vi "write data.vi"(8 "error in":errorcluster, 9 "timeout":i32=-1, 10 "data":string, 11 "lvlibretls connection in":refnum<class "lvlibretls connection.lvclass">) -> (0 "error out":errorcluster, 3 "lvlibretls connection out":refnum<class "lvlibretls connection.lvclass">)   [LabVIEW 2016, in "lvlibretls connection.lvclass"]
doc: "Writes all data to the network. Internally takes several attempts because libtls accepts only ~16 kB at a time (probably machine dependent). Trying to write a huge file will result in (a) many attempts, which could induce data copies, and (b) multiple \"string subset\" calls. Keeping writes under 10 kB where reasonable is a good idea unless you've really just got one big chunk of data (like an image). If you can process in smaller chunks (like sending a file off disk) you will probably see performance improvements from doing this."
uses:
  lvlibretls connection.lvclass
  lvlibretls connection.lvclass/lvlibretls connection.ctl
  tls library paths.vi
  lv tls dll.lvlib
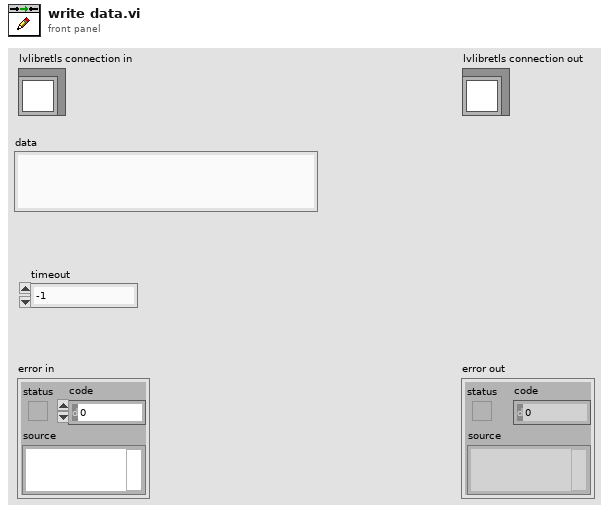
[diagram p1: front panel]
types:
  T1 = enum16{"Standard", "Buffered", "CRLF", "Immediate"}
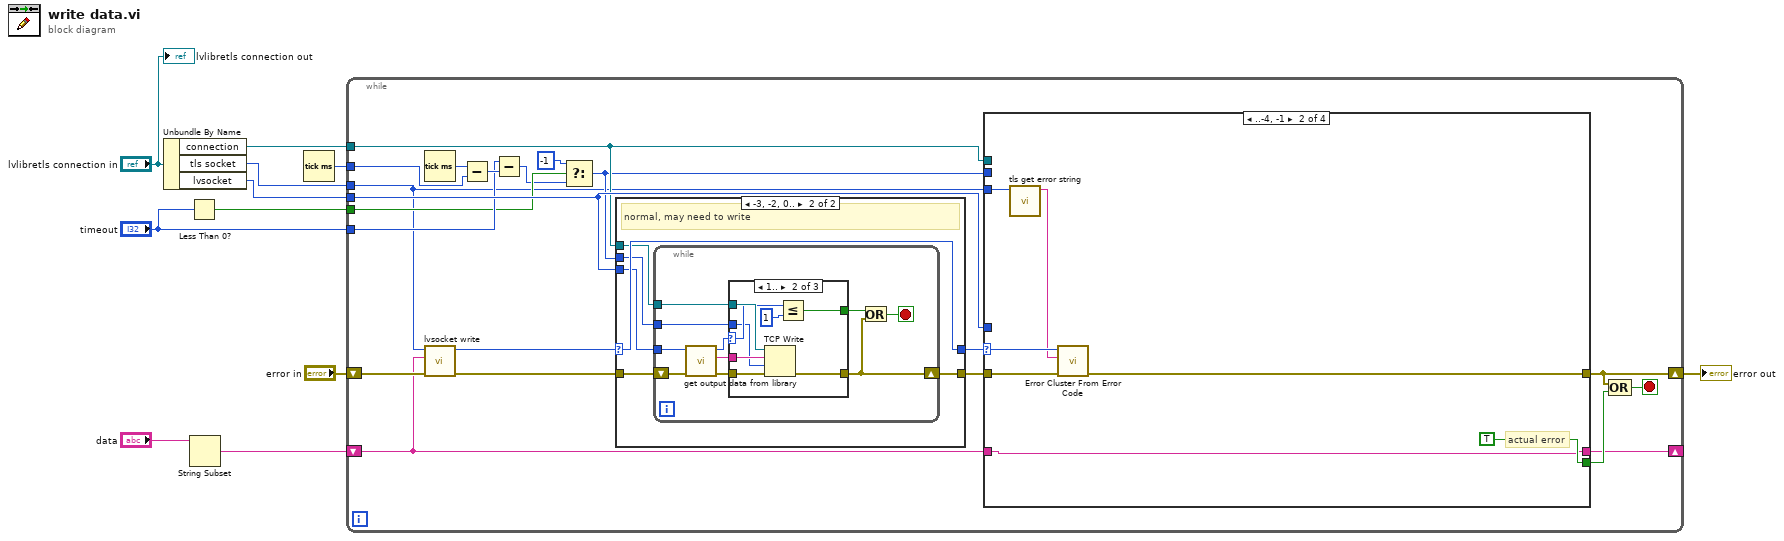
[diagram p0: block diagram]
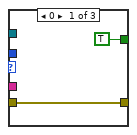
[diagram p3: hidden frame]
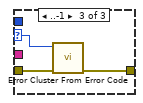
[diagram p4: hidden frame]
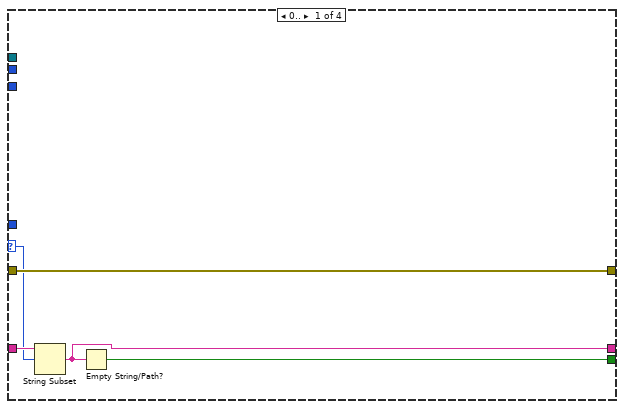
[diagram p5: hidden frame]
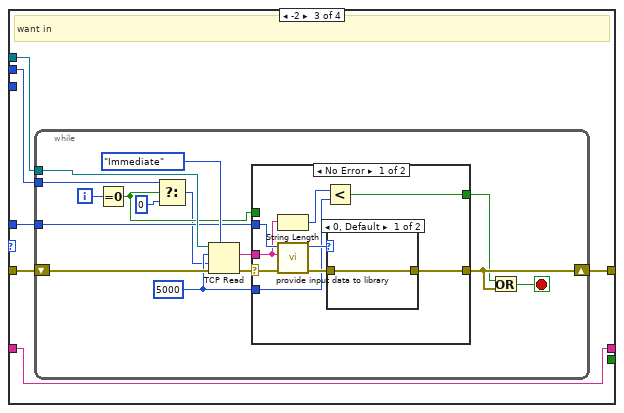
[diagram p6: hidden frame]
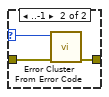
[diagram p7: hidden frame]
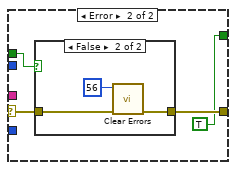
[diagram p8: hidden frame]
diagram:
  n1 = Unbundle By Name("lvlibretls connection in") -> ("connection"=w9:refnum<k5>, "tls socket"=w10:u64, "lvsocket"=w8:u64)
  n2 = Less Than 0?(x="timeout") -> (x < 0?=w4:bool)
  n3 = String Subset(string="data") -> (substring=w1:string)  [unwired: 2 in]
  n4 = Tick Count (ms)() -> (millisecond timer value=w3:u32)
  n5 = while {
    shift-right: [w31] -> w6
    shift-left: "error in" -> [w32]
    tunnel: w10 -> [w12]
    tunnel: w9 -> [w23]
    tunnel: w8 -> [w24]
    tunnel: "timeout" -> [w19]
    tunnel: w4 -> [w18]
    tunnel: w3 -> [w21]
    shift-right: [w13] -> _
    shift-left: w1 -> [w14]
    stop <- w30 stop-if-true
    n6 = Tick Count (ms)() -> (millisecond timer value=w22:u32)
    n7 = call "lvsocket write.vi"("error in"=w32, "data"=w14, "tls context"=w12) -> ("error out"=w25:errorcluster, "error response"=w28:i32)  [unwired: 7 in]
    n8 = Subtract(x=w22, y=w21) -> (x-y=w20:u32)
    n9 = Subtract(x=w19, y=w20) -> (x-y=w17:i32)
    n10 = Select(t=-1, s=w18, f=w17) -> (s? t:f=w15:i32)
    n11 = case shown="-3, -2, 0.." w28 {
      selector: w28 -> [w33 w40]
      tunnel: [w33 w40] -> w27
      tunnel: [w34 w38] -> w26
      tunnel: w25 -> [w34 w39]
      tunnel: w24 -> [_ w37]
      tunnel: w23 -> [_ w36]
      tunnel: w15 -> [_ w35]
      frame Default {
      }
      frame -3, -2, 0.. {
        # "normal, may need to write"
        n12 = while {
          shift-right: [w47] -> w38
          shift-left: w39 -> [w50]
          tunnel: w37 -> [w46]
          tunnel: w36 -> [w45]
          tunnel: w35 -> [w41]
          stop <- w44 stop-if-true
          n13 = call "get output data from library.vi"("error in"=w50, "lvsocket"=w46) -> ("error out"=w49:errorcluster, "data"=w42:string, "err"=w48:i32)  [unwired: 7 in]
          n14 = case shown="1.." w48 {
            selector: w48 -> [_ w56 w62]
            tunnel: w49 -> [w52 w60 w63]
            tunnel: [w52 w59 w61] -> w47
            tunnel: w42 -> [_ w58 _]
            tunnel: w45 -> [_ w57 _]
            tunnel: [TRUE w54 _] -> w43
            tunnel: w41 -> [_ w53 _]
            frame 0 {
            }
            frame 1.. {
              n15 = TCP Write(connection ID=w57, data in=w58, error in (no error)=w60, 9:w53) -> (error out=w59:errorcluster)  [unwired: 2 out]
              n16 = Less Or Equal?(x=w56, y=1) -> (x <= y?=w54:bool)
            }
            frame ..-1 {
              n17 = call <vilib>:"Error Cluster From Error Code.vi"("error in (no error)"=w63, "error code (0)"=w62) -> ("error out"=w61:errorcluster)  [unwired: 7 in]
            }
          }
          n18 = Or(x=w43, y=w47) -> (x .or. y?=w44:bool)
        }
      }
    }
    n19 = case shown="..-4, -1" w27 {
      selector: w27 -> [w66 w75 _ _]
      tunnel: [w68 w74 w79 w119] -> w31
      tunnel: [w64 TRUE _ _] -> w29
      tunnel: w23 -> [_ _ w81 _]
      tunnel: w24 -> [_ _ w80 _]
      tunnel: w26 -> [w68 w72 w78 w119]
      tunnel: w15 -> [_ _ w77 _]
      tunnel: w14 -> [w67 w71 w76 w118]
      tunnel: [w65 w71 w76 w118] -> w13
      tunnel: w12 -> [_ w70 _ _]
      frame 0.. {
        n20 = String Subset(string=w67, offset (0)=w66) -> (substring=w65:string)  [unwired: 1 in]
        n21 = Empty String/Path?(string/path=w65) -> (empty?=w64:bool)
      }
      frame ..-4, -1 {
        # "actual error"
        n22 = call "tls get error string.vi"("tls context"=w70) -> ("error string"=w69:string)  [unwired: 9 in, 1 out]
        n23 = call <vilib>:"Error Cluster From Error Code.vi"("error in (no error)"=w72, "error message (\"\")"=w69, "error code (0)"=w75) -> ("error out"=w74:errorcluster)  [unwired: 6 in]
      }
      frame -2 {
        # "want in"
        n24 = while {
          tunnel: w81 -> [w96]
          tunnel: w80 -> [w93]
          shift-right: [w91] -> w79
          shift-left: w78 -> [w92]
          tunnel: w77 -> [w84]
          i -> [w90]
          stop <- w89 stop-if-true
          w87 = 5000 ("bytes to read")
          n25 = Equal To 0?(x=w90) -> (x = 0?=w85:bool)
          n26 = Select(t=w84, s=w85, f=0 ("timeout ms (25000)")) -> (s? t:f=w82:i32)
          n27 = TCP Read(connection ID=w96, bytes to read=w87, error in (no error)=w92, 7:T1."Immediate" ("mode (standard)"), 9:w82) -> (data out=w86:string, error out=w94:errorcluster)  [unwired: 1 out]
          n28 = case shown="No Error" w94 {
            selector: w94 -> [w105 w113]
            tunnel: w86 -> [w97 _]
            tunnel: w93 -> [w98 _]
            tunnel: [w102 w112] -> w91
            tunnel: w85 -> [_ w111]
            tunnel: [w99 TRUE] -> w88
            tunnel: w87 -> [w100 _]
            frame No Error {
              n29 = String Length(string=w97) -> (length=w101:i32)
              n30 = call "provide input data to library.vi"("error in"=w105, "data in"=w97, "lvsocket"=w98) -> ("error out"=w104:errorcluster, "return"=w103:i32)  [unwired: 7 in]
              n31 = Less?(x=w101, y=w100) -> (x < y?=w99:bool)
              n32 = case shown="0, Default" w103 {
                selector: w103 -> [_ w108]
                tunnel: w104 -> [w106 w109]
                tunnel: [w106 w107] -> w102
                frame 0, Default {
                }
                frame ..-1 {
                  n33 = call <vilib>:"Error Cluster From Error Code.vi"("error in (no error)"=w109, "error code (0)"=w108) -> ("error out"=w107:errorcluster)  [unwired: 7 in]
                }
              }
            }
            frame Error {
              n34 = case shown="False" w111 {
                tunnel: w113 -> [w114 w117]
                tunnel: [w114 w116] -> w112
                frame True {
                }
                frame False {
                  n35 = call <vilib>:"Clear Errors.vi"("error in (no error)"=w117, "specific error code to clear (0: all)"=56) -> ("error out"=w116:errorcluster)  [unwired: 4 in, 1 out]
                }
              }
            }
          }
          n36 = Or(x=w88, y=w91) -> (x .or. y?=w89:bool)
        }
      }
      frame -3 {
        # "want out"
      }
    }
    n37 = Compound Arithmetic op=OR(w31, w29) -> (w30:bool)
  }
  "error out" <- w6
  "lvlibretls connection out" <- "lvlibretls connection in"
